vi "Terminate Condition Build Array.vi"(0 "Array in":dbl[][](array[numeric]), 1 "Reset Array?":bool, 3 "Start Analyzing Cycles at":u16=14, 5 "PLC Real-Time Clock (Min)":dbl, 7 "Disable 400 PPM Counter In":bool, 9 "Total Cycle Counter":u16, 11 "error in":errorcluster, 12 "Column 2":dbl, 14 "Column 3":dbl) -> (4 "Array out":dbl[][](array[numeric]), 8 "Disable 400 PPM Counter Our":bool, 15 "error out":errorcluster)   [LabVIEW 2023]
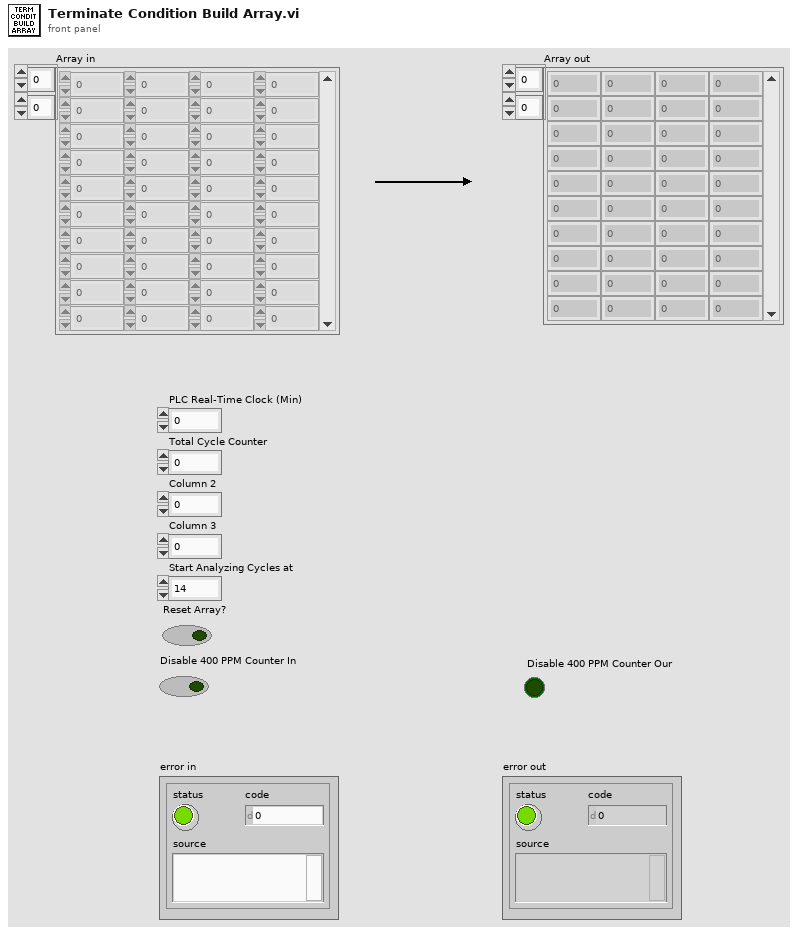
[diagram p1: front panel]
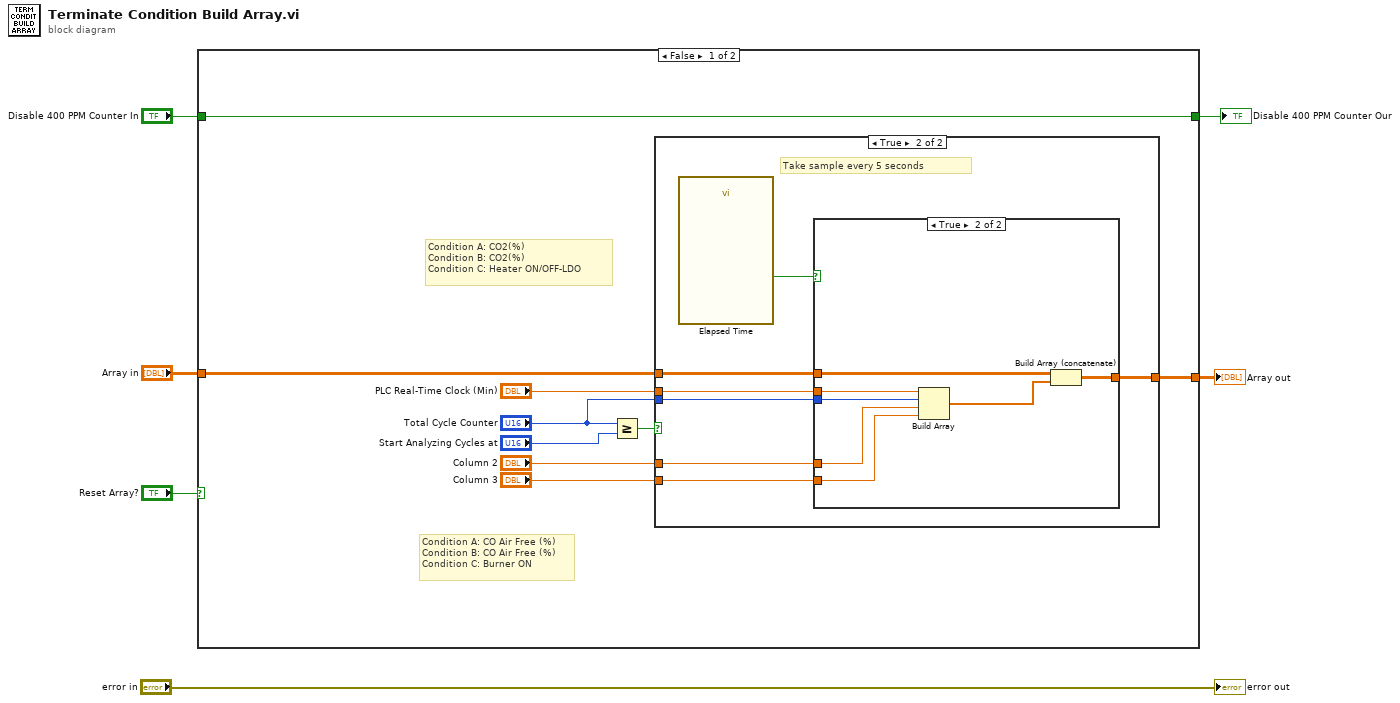
[diagram p0: block diagram]
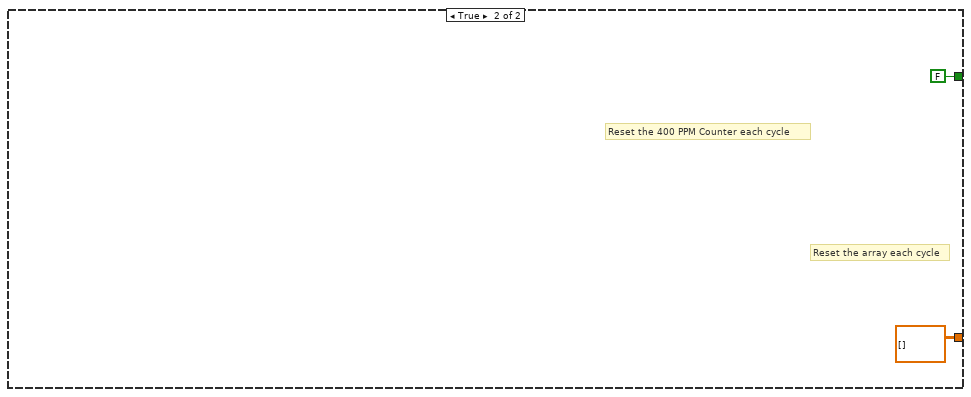
[diagram p4: hidden frame]
diagram:
  n1 = case shown="False" "Reset Array?" {
    tunnel: [w15 dbl[][] [] ("Array in")] -> w6
    tunnel: "Array in" -> [w14 _]
    tunnel: [w7 FALSE ("Disable 400 PPM Counter In")] -> w2
    tunnel: "Disable 400 PPM Counter In" -> [w7 _]
    frame False {
      # "Condition A: CO Air Free (%)\nCondition B: CO Air Free (%)\nCondition C: Burner ON"
      # "Condition A: CO2(%)\nCondition B: CO2(%)\nCondition C: Heater ON/OFF-LDO"
      n2 = Greater Or Equal?(x="Total Cycle Counter", y="Start Analyzing Cycles at") -> (x >= y?=w8:bool)
      n3 = case shown="True" w8 {
        tunnel: "PLC Real-Time Clock (Min)" -> [_ w23]
        tunnel: "Total Cycle Counter" -> [_ w22]
        tunnel: "Column 2" -> [_ w21]
        tunnel: "Column 3" -> [_ w20]
        tunnel: w14 -> [w16 w19]
        tunnel: [w16 w18] -> w15
        frame False {
        }
        frame True {
          # "Take sample every 5 seconds"
          n4 = call "Elapsed Time"() -> ("Time has Elapsed"=w17:bool)  [unwired: 12 in, 7 out]
          n5 = case shown="True" w17 {
            tunnel: w23 -> [_ w31]
            tunnel: w22 -> [_ w30]
            tunnel: w21 -> [_ w29]
            tunnel: w20 -> [_ w28]
            tunnel: w19 -> [w24 w26]
            tunnel: [w24 w25] -> w18
            frame False {
            }
            frame True {
              n6 = Build Array(w31, w30, w29, w28) -> (w27:dbl[])
              n7 = Build Array (concatenate)(w26, w27) -> (w25:dbl[][])
            }
          }
        }
      }
    }
    frame True {
      # "Reset the array each cycle"
      # "Reset the 400 PPM Counter each cycle"
    }
  }
  "Array out" <- w6
  "Disable 400 PPM Counter Our" <- w2
  "error out" <- "error in"
